vi "GVSDataView Add Graph VI.vi"(4 "DataView Idx":i32, 6 "Graph Main VIRef In":refnum<vi>, 7 "isFirstPanel":bool, 8 "Queue Name":string, 9 "GraphType":string="XY", 10 "panel_index":i32, 11 "Panel Ref In":refnum<vi>) -> (3 "bResult":bool)   [LabVIEW 2013]
uses:
  GVSNew View Global.vi
  SubVI/GVSData View Global.vi
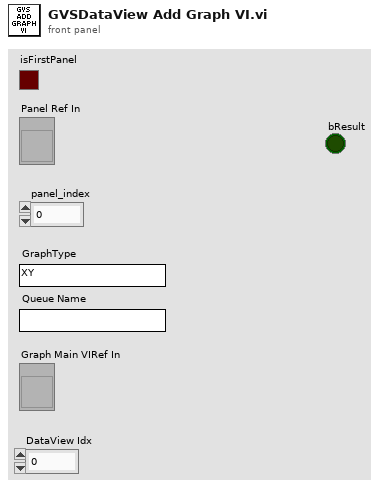
[diagram p1: front panel]
types:
  T1 = typedef "Graph Main Info Cluster.ctl" = cluster{"Selected_BarIdx":i32, "Selected_PanelIdx":i32, "Graph Main VIRef":refnum<vi>, "ToolBarClick":bool, "Spliter Ref Array":refnum<vi>[], "Panel Ref Array":refnum<vi>[], "Spliter_matrix":i32[][], "Panel_matrix":i32[][], "child_spliterIdx_matrix":i32[][], "split_pos_matrix":i32[][], "Title State":bool, "sQueueName":string, "Frame nID":i32, "Graph VIRef Array":cluster{"Graph VIRef":refnum<vi>, "Panel Idx":i32, "Frame VIRef":refnum<vi>, "Icon Ring":i32, "Graph Type":string}[], "View Type":string}
  T2 = cluster{"Graph VIRef":refnum<vi>, "Panel Idx":i32, "Frame VIRef":refnum<vi>, "Icon Ring":i32, "Graph Type":string}
  T3 = typedef "LVRectTypeDef.ctl" = cluster{"Left":i16, "Top":i16, "Right":i16, "Bottom":i16}
  T4 = typedef "GVSGraph Event.ctl" = cluster{"EvenName":string, "TitleName":string, "GraphName":string, "GraphType":string, "Data":variant, "Queue Name":string, "DataView Number":i32}
  T5 = cluster{"Graph VIRef":refnum<vi>, "Panel Idx":i32, "Frame VIRef":refnum<vi>, "Icon Ring":i32, "Graph Type":string}[]
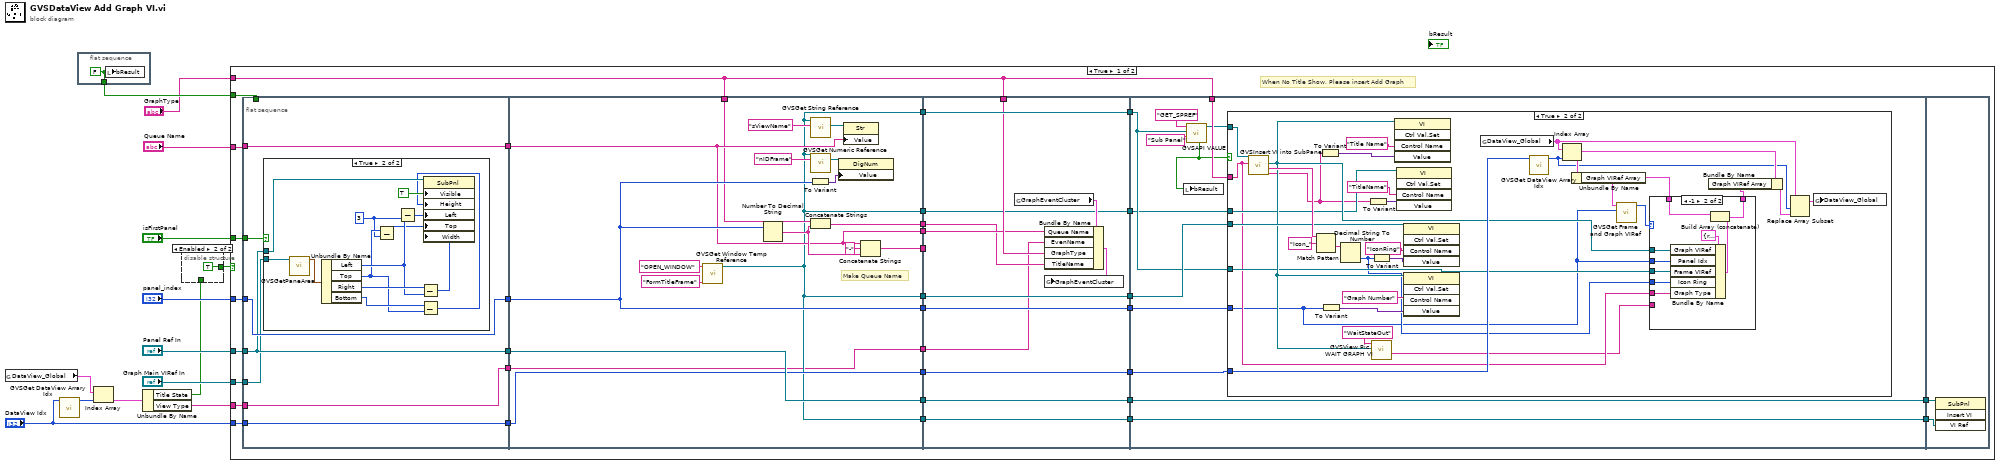
[diagram p0: block diagram]
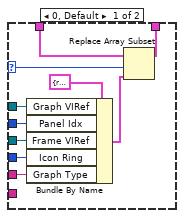
[diagram p5: hidden frame]
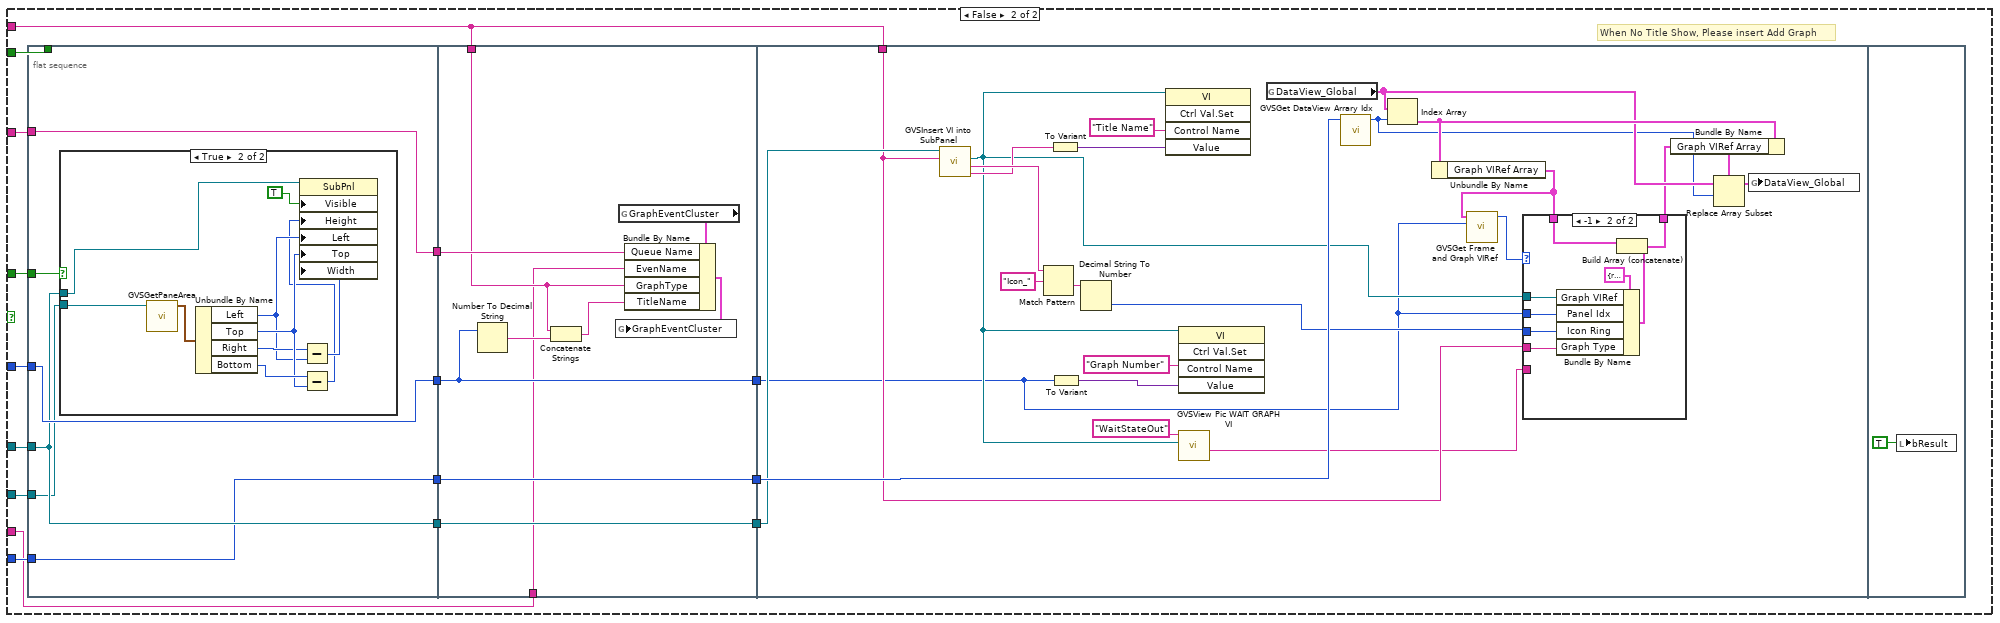
[diagram p6: hidden frame]
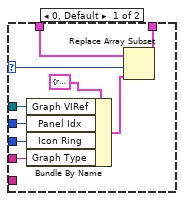
[diagram p8: hidden frame]
diagram:
  n1 = global read "GVSNew View Global.vi" "DataView_Global"() -> (w6:T1[])
  n2 = call "GVSGet DataView Arrary Idx.vi"("DataView Idx In"="DataView Idx") -> ("DataView Arrary Idx out"=w5:i32)  [unwired: 10 in]
  n3 = flat-sequence {
    tunnel: [w15] -> w9
    frame #0 {
      w15 = FALSE ("bResult")
      n4 = local write "bResult"(w15) -> ()
    }
  }
  n5 = Index Array(array=w6, index=w5) -> (element=w4:T1)
  n6 = Unbundle By Name(w4) -> ("Title State"=w2:bool, "View Type"=w3:string)
  n7 = disable-structure shown="Enabled" {
    disable-tunnel: w2 -> [w16 _]
    disable-tunnel: [w16 TRUE ("Title State")] -> w1
    frame Disabled {
    }
    frame Enabled {
    }
  }
  n8 = case shown="True" w1 {
    tunnel: "panel_index" -> [w28 w179]
    tunnel: "Panel Ref In" -> [w27 w178]
    tunnel: "Queue Name" -> [w26 w177]
    tunnel: "Graph Main VIRef In" -> [w25 w176]
    tunnel: "isFirstPanel" -> [w24 w175]
    tunnel: w9 -> [w23 w174]
    tunnel: "DataView Idx" -> [w22 w173]
    tunnel: "GraphType" -> [w21 w172]
    tunnel: w3 -> [w19 w167]
    frame True {
      # "When No Title Show, Please insert Add Graph"
      n9 = flat-sequence {
        tunnel: w27 -> [w55]
        tunnel: w26 -> [w57]
        tunnel: w28 -> [w58]
        tunnel: [w58] -> w51
        tunnel: [w57] -> w50
        tunnel: [w55] -> w49
        tunnel: w25 -> [w54]
        tunnel: w24 -> [w56]
        tunnel: w23 -> [_]
        tunnel: [w53] -> w48
        tunnel: w22 -> [w53]
        tunnel: [w52] -> w20
        tunnel: w19 -> [w52]
        tunnel: [w73] -> w47
        tunnel: w51 -> [w78]
        tunnel: w50 -> [w76]
        tunnel: w49 -> [w77]
        tunnel: [w82] -> w46
        tunnel: [w79] -> w45
        tunnel: [w73] -> w44
        tunnel: [w78] -> w43
        tunnel: [w77] -> w42
        tunnel: [w73] -> w41
        tunnel: [w76] -> w40
        tunnel: w48 -> [w75]
        tunnel: [w75] -> w39
        tunnel: w21 -> [w74]
        tunnel: [w73] -> w38
        tunnel: w20 -> [w72]
        tunnel: [w72] -> w18
        tunnel: w47 -> [w102]
        tunnel: [w102] -> w37
        tunnel: w21 -> [w99]
        tunnel: w46 -> [w92]
        tunnel: w45 -> [_]
        tunnel: [w98] -> w36
        tunnel: w44 -> [w98]
        tunnel: [w97] -> w35
        tunnel: w43 -> [w97]
        tunnel: [w96] -> w34
        tunnel: w42 -> [w96]
        tunnel: w41 -> [w95]
        tunnel: [w95] -> w33
        tunnel: w40 -> [w94]
        tunnel: [w93] -> w32
        tunnel: w39 -> [w93]
        tunnel: [w91] -> w31
        tunnel: w38 -> [w91]
        tunnel: w18 -> [w90]
        tunnel: w37 -> [w104]
        tunnel: w21 -> [w114]
        tunnel: w36 -> [w109]
        tunnel: w35 -> [w108]
        tunnel: [w107] -> w30
        tunnel: w34 -> [w107]
        tunnel: w33 -> [w106]
        tunnel: [w106] -> w29
        tunnel: w32 -> [w105]
        tunnel: w31 -> [w103]
        tunnel: w30 -> [w166]
        tunnel: w29 -> [w165]
        frame #0 {
          n10 = case shown="True" w56 {
            tunnel: w55 -> [_ w65]
            tunnel: w54 -> [_ w64]
            frame False {
            }
            frame True {
              w59 = i16 3 ("y")
              n11 = call "GVSGetPaneArea.vi"("vi reference"=w64) -> ("Content Area Rect"=w70:T3)  [unwired: 10 in]
              n12 = Unbundle By Name(w70) -> ("Left"=w67:i16, "Top"=w60:i16, "Right"=w68:i16, "Bottom"=w69:i16)
              n13 = Subtract(x=w60, y=w59) -> (x-y=w61:i16)
              n14 = Subtract(x=w67, y=w59) -> (x-y=w63:i16)
              n15 = Subtract(x=w68, y=w67) -> (x-y=w66:i16)
              n16 = Subtract(x=w69, y=w60) -> (x-y=w62:i16)
              n17 = property class="SubPnl"(reference=w65, "Visible"=TRUE, "Height"=w62, "Left"=w63, "Top"=w61, "Width"=w66) -> ()  [unwired: 1 in, 2 out]
            }
          }
        }
        frame #1 {
          # "Make Queue Name"
          n18 = call "GVSGet Window Temp Reference.vi"("sWindowName"="FormTitleFrame", "sAction"="OPEN_WINDOW") -> ("pVIRef_Out"=w73:refnum<vi>)  [unwired: 5 in, 4 out]
          n19 = Number To Decimal String(number=w78) -> (decimal integer string=w80:string)  [unwired: 1 in]
          n20 = To Variant(anything=w78) -> (Variant=w86:variant)
          n21 = call "GVSGet String Reference.vi"("Label Name"="sViewName", "VI Refnum"=w73) -> ("String Ref Out"=w88:refnum<vi>)  [unwired: 7 in, 2 out]
          n22 = call "GVSGet Numeric Reference.vi"("Label Name"="nIDFrame", "VI Refnum"=w73) -> ("Numeric Ref Out"=w87:refnum<vi>)  [unwired: 7 in, 2 out]
          n23 = Concatenate Strings(w74, w80) -> (w82:string)
          n24 = property class="DigNum"(reference=w87, "Value"=w86) -> ()  [unwired: 1 in, 2 out]
          n25 = property class="Str"(reference=w88, "Value"=w76) -> ()  [unwired: 1 in, 2 out]
          n26 = Concatenate Strings(w76, "-" ("string"), w80) -> (w79:string)
        }
        frame #2 {
          n27 = global read "GVSData View Global.vi" "GraphEventCluster"() -> (w101:T4)
          n28 = Bundle By Name(cluster=w101, "Queue Name"=w94, "EvenName"=w90, "GraphType"=w99, "TitleName"=w92) -> (w100:T4)
          n29 = global write "GVSData View Global.vi" "GraphEventCluster"(w100) -> ()
        }
        frame #3 {
          n30 = call "GVSAPI VALUE.vi"("sControlName"="Sub Panel", "pVIRef"=w104, "sAction"="GET_SPREF") -> ("pSPRef"=w111:refnum<vi>, "bResult"=w110:bool)  [unwired: 4 in, 3 out]
          n31 = local write "bResult"(w110) -> ()
          n32 = case shown="True" w110 {
            tunnel: w114 -> [_ w119]
            tunnel: w111 -> [_ w145]
            tunnel: w109 -> [_ w139]
            tunnel: w108 -> [_ w117]
            tunnel: w105 -> [_ w135]
            tunnel: w104 -> [_ w127]
            tunnel: w103 -> [_ w124]
            frame False {
            }
            frame True {
              n33 = call "GVSInsert VI into SubPanel.vi"("WindowType"=w119, "SubPanel Ref"=w145) -> ("WindowName"=w121:string, "Icon Out"=w140:string, "VI Ref Out"=w128:refnum<vi>)  [unwired: 6 in, 1 out]
              n34 = Match Pattern(string=w140, regular expression="Icon_") -> (after substring=w144:string)  [unwired: 1 in, 3 out]
              n35 = To Variant(anything=w121) -> (Variant=w126:variant)
              n36 = To Variant(anything=w117) -> (Variant=w137:variant)
              n37 = Decimal String To Number(string=w144) -> (number=w120:i32)  [unwired: 2 in, 1 out]
              n38 = To Variant(anything=w121) -> (Variant=w123:variant)
              n39 = call "GVSView Pic WAIT GRAPH VI.vi"("vi reference"=w128, "sAction"="WaitStateOut") -> ("sData_Out"=w115:string)  [unwired: 9 in]
              n40 = To Variant(anything=w120) -> (Variant=w141:variant)
              n41 = invoke class="VI" method="Ctrl Val.Set"(reference=w128, "Control Name"="Title Name" ("Label Name"), "Value"=w126) -> ()  [unwired: 2 in, 5 out]
              n42 = invoke class="VI" method="Ctrl Val.Set"(reference=w124, "Control Name"="TitleName" ("Label Name"), "Value"=w123) -> ()  [unwired: 2 in, 5 out]
              n43 = invoke class="VI" method="Ctrl Val.Set"(reference=w139, "Control Name"="IconRing", "Value"=w141) -> ()  [unwired: 2 in, 5 out]
              n44 = invoke class="VI" method="Ctrl Val.Set"(reference=w128, "Control Name"="Graph Number", "Value"=w137) -> ()  [unwired: 2 in, 5 out]
              n45 = global read "GVSNew View Global.vi" "DataView_Global"() -> (w132:T1[])
              n46 = call "GVSGet DataView Arrary Idx.vi"("DataView Idx In"=w135) -> ("DataView Arrary Idx out"=w131:i32)  [unwired: 10 in]
              n47 = Index Array(array=w132, index=w131) -> (element=w134:T1)
              n48 = Unbundle By Name(w134) -> ("Graph VIRef Array"=w118:T5)
              n49 = call "GVSGet Frame and Graph VIRef.vi"("Panel Idx"=w117, "Graph VIRef Array"=w118) -> ("Graph VIRef Array Index"=w116:i32)  [unwired: 5 in, 4 out]
              n50 = case shown="-1" w116 {
                selector: w116 -> [w153 _]
                tunnel: w118 -> [w155 w164]
                tunnel: [w154 w162] -> w133
                tunnel: w128 -> [w152 w161]
                tunnel: w117 -> [w151 w160]
                tunnel: w127 -> [w150 w159]
                tunnel: w120 -> [w149 w158]
                tunnel: w119 -> [w148 w156]
                tunnel: w115 -> [_ _]
                frame 0, Default {
                  n51 = Bundle By Name(cluster=T2 {"Graph VIRef"=refnum, "Panel Idx"=0, "Frame VIRef"=refnum, "Icon Ring"=0, "Graph Type"=""} ("element"), "Graph VIRef"=w152, "Panel Idx"=w151, "Frame VIRef"=w150, "Icon Ring"=w149, "Graph Type"=w148) -> (w146:T2)
                  n52 = Replace Array Subset(array=w155, new element=w146, index=w153) -> (w154:T5)
                }
                frame -1 {
                  n53 = Bundle By Name(cluster=T2 {"Graph VIRef"=refnum, "Panel Idx"=0, "Frame VIRef"=refnum, "Icon Ring"=0, "Graph Type"=""} ("element"), "Graph VIRef"=w161, "Panel Idx"=w160, "Frame VIRef"=w159, "Icon Ring"=w158, "Graph Type"=w156) -> (w163:T2)
                  n54 = Build Array (concatenate)(w164, w163) -> (w162:T5)
                }
              }
              n55 = Bundle By Name(cluster=w134, "Graph VIRef Array"=w133) -> (w130:T1)
              n56 = Replace Array Subset(array=w132, new element=w130, index=w131) -> (w129:T1[])
              n57 = global write "GVSNew View Global.vi" "DataView_Global"(w129) -> ()
            }
          }
        }
        frame #4 {
          n58 = invoke class="SubPnl" method="Insert VI"(reference=w166, "VI Ref"=w165) -> ()  [unwired: 2 in, 4 out]
        }
      }
    }
    frame False {
      # "When No Title Show, Please insert Add Graph"
      n59 = flat-sequence {
        tunnel: w178 -> [w185]
        tunnel: w177 -> [w187]
        tunnel: w179 -> [w188]
        tunnel: [w188] -> w171
        tunnel: [w187] -> w170
        tunnel: [w185] -> w169
        tunnel: w176 -> [w184]
        tunnel: w175 -> [w186]
        tunnel: w174 -> [_]
        tunnel: [w183] -> w168
        tunnel: w173 -> [w183]
        tunnel: w172 -> [w202]
        tunnel: [w201] -> w182
        tunnel: w171 -> [w201]
        tunnel: [w206] -> w181
        tunnel: w169 -> [w206]
        tunnel: w170 -> [w205]
        tunnel: [w204] -> w180
        tunnel: w168 -> [w204]
        tunnel: w167 -> [w199]
        tunnel: w172 -> [w213]
        tunnel: w182 -> [w210]
        tunnel: w181 -> [w231]
        tunnel: w180 -> [w232]
        frame #0 {
          n60 = case shown="True" w186 {
            tunnel: w185 -> [_ w190]
            tunnel: w184 -> [_ w189]
            frame False {
            }
            frame True {
              n61 = call "GVSGetPaneArea.vi"("vi reference"=w189) -> ("Content Area Rect"=w197:T3)  [unwired: 10 in]
              n62 = Unbundle By Name(w197) -> ("Left"=w193:i16, "Top"=w195:i16, "Right"=w194:i16, "Bottom"=w196:i16)
              n63 = Subtract(x=w194, y=w193) -> (x-y=w192:i16)
              n64 = Subtract(x=w196, y=w195) -> (x-y=w191:i16)
              n65 = property class="SubPnl"(reference=w190, "Visible"=TRUE, "Height"=w191, "Left"=w193, "Top"=w195, "Width"=w192) -> ()  [unwired: 1 in, 2 out]
            }
          }
        }
        frame #1 {
          n66 = Number To Decimal String(number=w201) -> (decimal integer string=w203:string)  [unwired: 1 in]
          n67 = Concatenate Strings(w202, w203) -> (w200:string)
          n68 = global read "GVSData View Global.vi" "GraphEventCluster"() -> (w208:T4)
          n69 = Bundle By Name(cluster=w208, "Queue Name"=w205, "EvenName"=w199, "GraphType"=w202, "TitleName"=w200) -> (w207:T4)
          n70 = global write "GVSData View Global.vi" "GraphEventCluster"(w207) -> ()
        }
        frame #2 {
          n71 = call "GVSInsert VI into SubPanel.vi"("WindowType"=w213, "SubPanel Ref"=w231) -> ("WindowName"=w217:string, "Icon Out"=w228:string, "VI Ref Out"=w215:refnum<vi>)  [unwired: 6 in, 1 out]
          n72 = Match Pattern(string=w228, regular expression="Icon_") -> (after substring=w230:string)  [unwired: 1 in, 3 out]
          n73 = To Variant(anything=w217) -> (Variant=w219:variant)
          n74 = To Variant(anything=w210) -> (Variant=w226:variant)
          n75 = Decimal String To Number(string=w230) -> (number=w214:i32)  [unwired: 2 in, 1 out]
          n76 = invoke class="VI" method="Ctrl Val.Set"(reference=w215, "Control Name"="Title Name" ("Label Name"), "Value"=w219) -> ()  [unwired: 2 in, 5 out]
          n77 = invoke class="VI" method="Ctrl Val.Set"(reference=w215, "Control Name"="Graph Number", "Value"=w226) -> ()  [unwired: 2 in, 5 out]
          n78 = call "GVSView Pic WAIT GRAPH VI.vi"("vi reference"=w215, "sAction"="WaitStateOut") -> ("sData_Out"=w209:string)  [unwired: 9 in]
          n79 = global read "GVSNew View Global.vi" "DataView_Global"() -> (w223:T1[])
          n80 = call "GVSGet DataView Arrary Idx.vi"("DataView Idx In"=w232) -> ("DataView Arrary Idx out"=w222:i32)  [unwired: 10 in]
          n81 = Index Array(array=w223, index=w222) -> (element=w224:T1)
          n82 = Unbundle By Name(w224) -> ("Graph VIRef Array"=w211:T5)
          n83 = call "GVSGet Frame and Graph VIRef.vi"("Panel Idx"=w210, "Graph VIRef Array"=w211) -> ("Graph VIRef Array Index"=w216:i32)  [unwired: 5 in, 4 out]
          n84 = case shown="-1" w216 {
            selector: w216 -> [w239 _]
            tunnel: w211 -> [w241 w249]
            tunnel: [w240 w247] -> w212
            tunnel: w215 -> [w238 w246]
            tunnel: w210 -> [w237 w245]
            tunnel: w214 -> [w236 w242]
            tunnel: w213 -> [w235 w243]
            tunnel: w209 -> [_ _]
            frame 0, Default {
              n85 = Bundle By Name(cluster=T2 {"Graph VIRef"=refnum, "Panel Idx"=0, "Frame VIRef"=refnum, "Icon Ring"=0, "Graph Type"=""} ("element"), "Graph VIRef"=w238, "Panel Idx"=w237, "Icon Ring"=w236, "Graph Type"=w235) -> (w233:T2)
              n86 = Replace Array Subset(array=w241, new element=w233, index=w239) -> (w240:T5)
            }
            frame -1 {
              n87 = Bundle By Name(cluster=T2 {"Graph VIRef"=refnum, "Panel Idx"=0, "Frame VIRef"=refnum, "Icon Ring"=0, "Graph Type"=""} ("element"), "Graph VIRef"=w246, "Panel Idx"=w245, "Icon Ring"=w242, "Graph Type"=w243) -> (w248:T2)
              n88 = Build Array (concatenate)(w249, w248) -> (w247:T5)
            }
          }
          n89 = Bundle By Name(cluster=w224, "Graph VIRef Array"=w212) -> (w221:T1)
          n90 = Replace Array Subset(array=w223, new element=w221, index=w222) -> (w220:T1[])
          n91 = global write "GVSNew View Global.vi" "DataView_Global"(w220) -> ()
        }
        frame #3 {
          n92 = local write "bResult"(TRUE ("bResult")) -> ()
        }
      }
    }
  }
